vi "FindSubpanelIfActive.vi"(8 "error in (no error)":errorcluster, 10 "EmbeddedSMO in":refnum<class "SMO.UI.Embedded.lvclass">, 11 "SMO.UI.MAUI in":refnum<class "SMO.UI.MAUI.lvclass">) -> (0 "error out":errorcluster, 1 "Panel":T1, 2 "Found?":bool, 3 "SMO.UI.MAUI out":refnum<class "SMO.UI.MAUI.lvclass">, 4 "Panel Index":i32)   [LabVIEW 2016, in "SMO.UI.MAUI.lvclass"]
uses:
  SMO.UI.MAUI.lvclass
  <vilib>/Levylab/SMO.UI.Embedded/SMO.UI.Embedded.lvclass
  C:/Program Files (x86)/National Instruments/LabVIEW 2016/vi.lib/JKI/JKI SMO/SMO/SMO.lvclass
  Typedefs/PanelData.ctl
  SMO.UI.MAUI.lvclass/SMO.UI.MAUI.ctl
  <vilib>/JKI/JKI SMO/SMO/SMO.lvclass
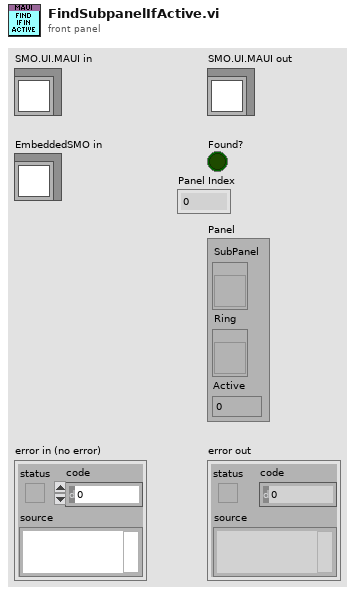
[diagram p1: front panel]
types:
  T1 = typedef "SMO.UI.MAUI.lvclass/PanelData.ctl" = cluster{"SubPanel":refnum<vi>, "Ring":refnum<vi>, "Active":i32}
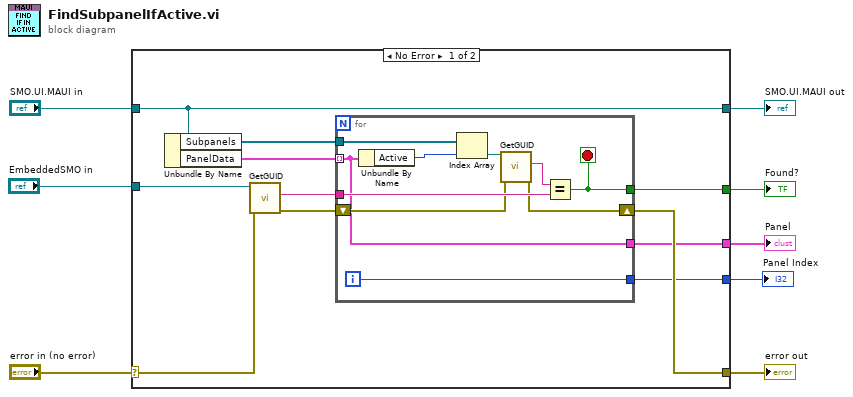
[diagram p0: block diagram]
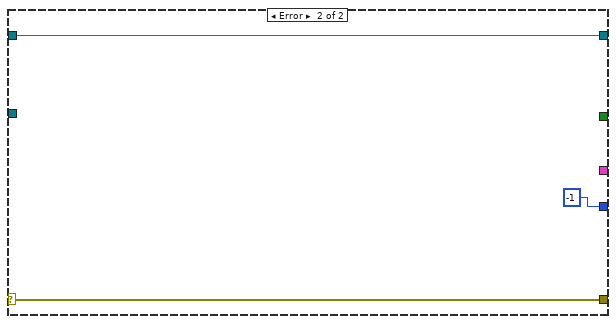
[diagram p2: hidden frame]
diagram:
  n1 = case shown="No Error" "error in (no error)" {
    selector: "error in (no error)" -> [w12 w32]
    tunnel: [w13 w32] -> w7
    tunnel: [w19 w31] -> w5
    tunnel: "SMO.UI.MAUI in" -> [w19 w31]
    tunnel: "EmbeddedSMO in" -> [w16 _]
    tunnel: [w11 _] -> w3
    tunnel: [w10 _] -> w2
    tunnel: [w9 -1] -> w1
    frame No Error {
      n2 = Unbundle By Name(w19) -> ("Subpanels"=w18:refnum<class "SMO.UI.Embedded.lvclass">[], "PanelData"=w17:T1[])
      n3 = call <vilib>:"GetGUID.vi"("error in (no error)"=w12, "SMO"=w16) -> ("error out"=w14:errorcluster, "GUID"=w15:string)  [unwired: 7 in, 1 out]
      n4 = for {
        tunnel: w18 -> [w28]
        tunnel: w17 -> [w21] mode=indexing
        tunnel: w15 -> [w25]
        tunnel: [w24] -> w11
        shift-right: [w22] -> w13
        shift-left: w14 -> [w23]
        tunnel: [w21] -> w10
        tunnel: [w20] -> w9
        i -> [w20]
        stop <- w24 stop-if-true
        n5 = Unbundle By Name(w21) -> ("Active"=w29:i32)
        n6 = Index Array(array=w28, index=w29) -> (element=w27:refnum<class "SMO.UI.Embedded.lvclass">)
        n7 = call <vilib>:"GetGUID.vi"("error in (no error)"=w23, "SMO"=w27) -> ("error out"=w22:errorcluster, "GUID"=w26:string)  [unwired: 7 in, 1 out]
        n8 = Equal?(x=w26, y=w25) -> (x = y?=w24:bool)
      }
    }
    frame Error {
    }
  }
  "error out" <- w7
  "SMO.UI.MAUI out" <- w5
  "Found?" <- w3
  "Panel" <- w2
  "Panel Index" <- w1
